vi "drive arctan.vi"(1 "x/y (tan)":fxp<+/-,32,16>) -> (0 "Numeric 2":i8)   [LabVIEW 2010]
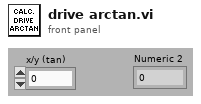
[diagram p1: front panel]
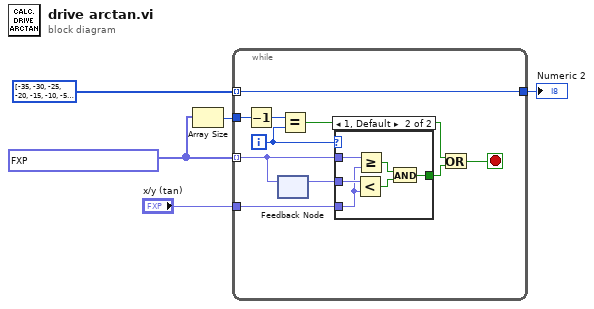
[diagram p0: block diagram]
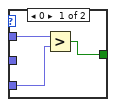
[diagram p2: hidden frame]
diagram:
  w1 = fxp<+/-,16,1>[] [-0.7001953125, -0.577362060546875, -0.46630859375, -0.363983154296875, -0.2679443359375, -0.17633056640625, -0.087493896484375, 0.0, -0.0174560546875, 0.0174560546875, 0.17633056640625, 0.2679443359375, 0.363983154296875, 0.46630859375, 0.577362060546875, 0.7001953125, 0.0, 0.0, 0.0, 0.0, 0.0, 0.0, 0.0, 0.0, 0.0, 0.0, 0.0, 0.0, 0.0, 0.0, 0.0, 0.0, 0.0, 0.0, 0.0, 0.0, 0.0, 0.0, 0.0, 0.0, 0.0, 0.0, 0.0, 0.0, 0.0, 0.0, 0.0, 0.0, 0.0, 0.0, 0.0, 0.0, 0.0, 0.0, 0.0, 0.0, 0.0, 0.0, 0.0, 0.0, 0.0, 0.0, 0.0, 0.0, 0.0, 0.0, 0.0, 0.0, 0.0, 0.0, 0.0, 0.0, 0.0, 0.0, 0.0, 0.0, 0.0, 0.0, 0.0, 0.0, 0.0, 0.0, 0.0, 0.0, 0.0, 0.0, 0.0, 0.0, 0.0, 0.0, 0.0, 0.0, 0.0, 0.0, 0.0, 0.0, 0.0, 0.0, 0.0, 0.0, 0.0, 0.0, 0.0, 0.0, 0.0, 0.0, 0.0, 0.0, 0.0, 0.0, 0.0, 0.0, 0.0, 0.0, 0.0, 0.0, 0.0, 0.0, 0.0, 0.0, 0.0, 0.0, 0.0, 0.0, 0.0, 0.0, 0.0, 0.0, 0.0, 0.0, 0.0, 0.0, 0.0, 0.0, 0.0, 0.0, 0.0, 0.0, 0.0, 0.0, 0.0, 0.0, 0.0, 0.0, 0.0, 0.0, 0.0, 0.0, 0.0, 0.0, 0.0, 0.0, 0.0, 0.0, 0.0, 0.0, 0.0, 0.0, 0.0, 0.0, 0.0, 0.0, 0.0, 0.0, 0.0, 0.0, 0.0, 0.0, 0.0, 0.0, 0.0, 0.0, 0.0, 0.0, 0.0, 0.0, 0.0, 0.0, 0.0, 0.0, 0.0, 0.0, 0.0, 0.0, 0.0, 0.0, 0.0, 0.0, 0.0, 0.0, 0.0, 0.0, 0.0, 0.0, 0.0, 0.0, 0.0, 0.0, 0.0, 0.0, 0.0, 0.0, 0.0, 0.0, 0.0, 0.0, 0.0, 0.0, 0.0, 0.0, 0.0, 0.0, 0.0, 0.0, 0.0, 0.0, 0.0, 0.0, 0.0, 0.0, 0.0, 0.0, 0.0, 0.0, 0.0, 0.0, 0.0, 0.0, 0.0, 0.0, 0.0, 0.0, 0.0, 0.0, 0.0, 0.0, 0.0, 0.0, 0.0, 0.0, 0.0, 0.0, 0.0, 0.0, 0.0, 0.0, 0.0, 0.0, 0.0, 0.0, 0.0, 0.0, 0.0, 0.0, 0.0, 0.0, 0.0, 0.0, 0.0, 0.0, 0.0, 0.0, 0.0, 0.0, 0.0, 0.0, 0.0, 0.0, 0.0, 0.0, 0.0, 0.0, 0.0, 0.0, 0.0, 0.0, 0.0, 0.0, 0.0, 0.0, 0.0, 0.0, 0.0, 0.0, 0.0, 0.0, 0.0, 0.0, 0.0, 0.0, 0.0, 0.0, 0.0, 0.0, 0.0, 0.0, 0.0, 0.0, 0.0, 0.0, 0.0, 0.0, 0.0, 0.0, 0.0, 0.0, 0.0, 0.0, 0.0, 0.0, 0.0, 0.0, 0.0, 0.0, 0.0, 0.0, 0.0, 0.0, 0.0, 0.0, 0.0, 0.0, 0.0, 0.0, 0.0, 0.0, 0.0, 0.0, 0.0, 0.0, 0.0, 0.0, 0.0, 0.0, 0.0, 0.0, 0.0, 0.0, 0.0, 0.0, 0.0, 0.0, 0.0, 0.0, 0.0, 0.0, 0.0, 0.0, 0.0, 0.0, 0.0, 0.0, 0.0, 0.0, 0.0, 0.0, 0.0, 0.0, 0.0, 0.0, 0.0, 0.0] ("Modified Tangent")
  n1 = Array Size(array=w1) -> (size(s)=w4:i32)
  n2 = while {
    tunnel: w1 -> [w8] mode=indexing
    tunnel: "x/y (tan)" -> [w14]
    tunnel: w4 -> [w12]
    tunnel: [w6] -> w3
    tunnel: i8[] [-35, -30, -25, -20, -15, -10, -5, -1, 1, 5, 10, 15, 20, 25, 30, 35] -> [w6] mode=indexing
    i -> [w7]
    stop <- w9 stop-if-true
    n3 = Decrement(x=w12) -> (x-1=w11:i32)
    n4 = feedback-in #1(w8) -> ()
    n5 = feedback #1() -> (w15:fxp<+/-,16,1>)  [unwired: 1 in]
    n6 = Equal?(x=w11, y=w7) -> (x = y?=w10:bool)
    n7 = case shown="1, Default" w7 {
      tunnel: w15 -> [_ w24]
      tunnel: w14 -> [w16 w23]
      tunnel: [w18 w20] -> w13
      tunnel: w8 -> [w17 w19]
      frame 0 {
        n8 = Greater?(x=w17, y=w16) -> (0:w18:bool)
      }
      frame 1, Default {
        n9 = Less?(x=w24, y=w23) -> (x < y?=w22:bool)
        n10 = Greater Or Equal?(x=w19, y=w23) -> (x >= y?=w21:bool)
        n11 = And(x=w21, y=w22) -> (x .and. y?=w20:bool)
      }
    }
    n12 = Or(x=w10, y=w13) -> (x .or. y?=w9:bool)
  }
  "Numeric 2" <- w3
